vi "CL_Post-process_timestamps.vi"(6 "Timing calibration sw/hw":dbl, 8 "Start time (SW)":timestamp, 9 "Start time (HW)":u32, 10 "HW timestamp and delta in":u32[][](array[numeric]), 11 "SW timestamp in":dbl[](array[numeric])) -> (2 "HW timestamp and delta out":u32[][](array[numeric]), 3 "SW timestamp out":dbl[](array[numeric]))   [LabVIEW 2018, in "Tracker.lvlib"]
uses:
  Tracker.lvlib
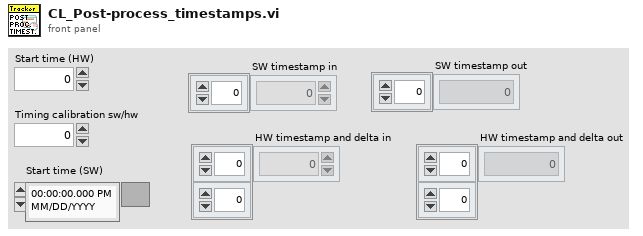
[diagram p1: front panel]
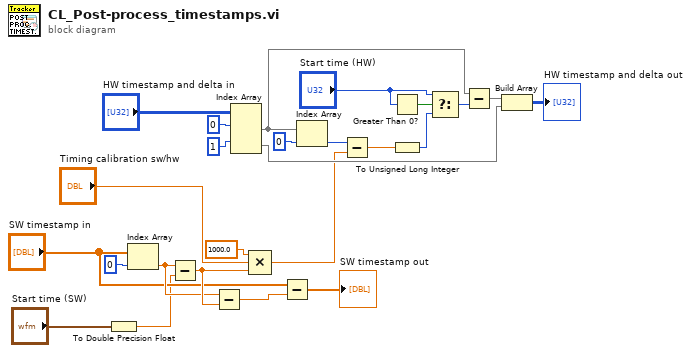
[diagram p0: block diagram]
diagram:
  n1 = To Double Precision Float(number="Start time (SW)") -> (double precision float=w6:dbl)
  n2 = Index Array(array="SW timestamp in", index=0) -> (element=w16:dbl)
  n3 = Subtract(x=w16, y=w6) -> (x-y=w17:dbl)
  n4 = Subtract(x=w16, y=w17) -> (x-y=w18:dbl)
  n5 = Index Array(array="HW timestamp and delta in", index (row) #1=0 ("index (row)"), index (row) #2=1 ("index (row)")) -> (element #1=w20:u32[], element #2=w24:u32[])  [unwired: 2 in]
  n6 = Compound Arithmetic op=MULTIPLY(1000.0 ("value"), "Timing calibration sw/hw", w17) -> (w12:dbl)
  n7 = Subtract(x="SW timestamp in", y=w18) -> (x-y=→"SW timestamp out":dbl[])
  n8 = Index Array(array=w20, index=0) -> (element=w11:u32)
  n9 = Subtract(x=w11, y=w12) -> (x-y=w13:dbl)
  n10 = Greater Than 0?(x="Start time (HW)") -> (x > 0?=w2:bool)
  n11 = To Unsigned Long Integer(number=w13) -> (unsigned 32bit integer=w21:u32)
  n12 = Select(t="Start time (HW)", s=w2, f=w21) -> (s? t:f=w1:u32)
  n13 = Subtract(x=w20, y=w1) -> (x-y=w23:u32[])
  n14 = Build Array(w23, w24) -> (→"HW timestamp and delta out":u32[][])
